vi "Wait till all GFG events stop_for fixed duration.vi"(8 "error in (no error)":errorcluster) -> (0 "error out":errorcluster)   [LabVIEW 2012]
doc: "SciScan 1.2 160622"
uses:
  <vilib>/Utility/VariantDataType/Type.ctl
  <vilib>/Utility/VariantDataType/VariantType.lvlib
panel:
  out "Array":T1(array[cluster])
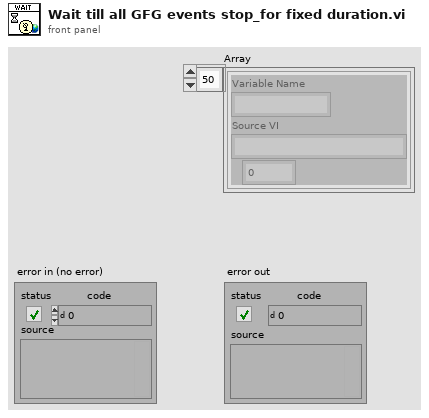
[diagram p1: front panel]
types:
  T1 = cluster{"Variable Name":string, "Source VI":string, u32}[]
  T2 = cluster{"Variable Name":string, "Source VI":string, u32}
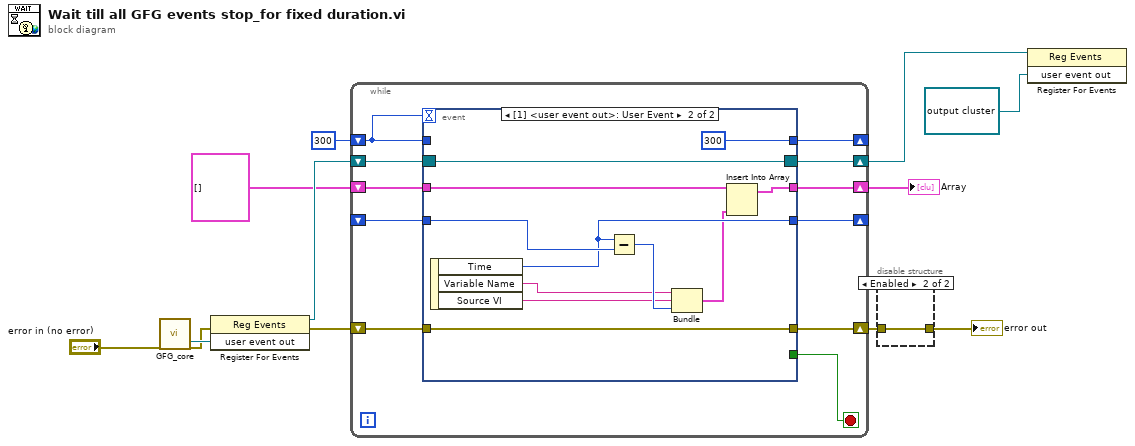
[diagram p0: block diagram]
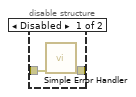
[diagram p2: hidden frame]
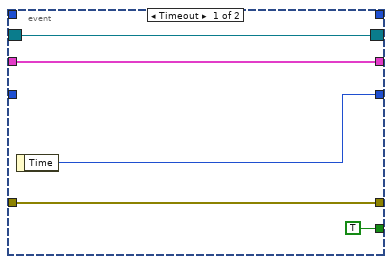
[diagram p3: hidden frame]
diagram:
  n1 = call "GFG_core.vi"("error in (no error)"="error in (no error)") -> ("user event out"=w2:refnum<user-event>, "error out"=w1:errorcluster)  [unwired: 12 in, 5 out]
  n2 = register-events(error in=w1, w2) -> (reference out=w12:refnum<event-registration>, error out=w9:errorcluster)  [unwired: 1 in]
  n3 = while {
    shift-right: [w22] -> _
    shift-left: 300 -> [w16]
    shift-right: [w20] -> _
    shift-left: _ -> [w19]
    shift-right: [w17] -> w6
    shift-left: w9 -> [w18]
    shift-right: [w15] -> w4
    shift-left: w12 -> [w23]
    shift-right: [w13] -> w7
    shift-left: T1 [] -> [w14]
    stop <- w21 stop-if-true
    n4 = event shown="[1] <user event out>: User Event" {
      selector: w23 -> [w26 w32]
      dyn-events: [w26 w32] -> w15
      timeout: w16 -> [_ _]
      tunnel: [_ 300] -> w22
      tunnel: [TRUE _] -> w21
      tunnel: [w25 w37] -> w20
      tunnel: w19 -> [_ w38]
      tunnel: w18 -> [w27 w35]
      tunnel: [w27 w35] -> w17
      tunnel: w16 -> [_ _]
      tunnel: w14 -> [w24 w31]
      tunnel: [w24 w29] -> w13
      event Timeout {
        n5 = event-data() -> ("Time"=w25:u32)  [unwired: 1 in]
      }
      event User Event {
        n6 = event-data() -> ("Time"=w37:u32, "Variable Name"=w33:string, "Source VI"=w34:string)  [unwired: 1 in]
        n7 = Subtract(x=w37, y=w38) -> (x-y=w36:u32)
        n8 = Bundle("Variable Name"=w33, "Source VI"=w34, w36) -> (w30:T2)  [unwired: 1 in]
        n9 = Insert Into Array(array=w31, new element=w30) -> (w29:T1)  [unwired: 1 in]
      }
    }
  }
  "Array" <- w7
  n10 = disable-structure shown="Enabled" {
    disable-tunnel: w6 -> [w41 w42]
    disable-tunnel: [w40 w42] -> w5
    frame Disabled {
      n11 = call <vilib>:"Simple Error Handler.vi"("error in (no error)"=w41) -> ("error out"=w40:errorcluster)  [unwired: 4 in, 4 out]
    }
    frame Enabled {
    }
  }
  "error out" <- w5
  n12 = register-events(reference=w4, refnum<user-event> refnum ("event source")) -> ()  [unwired: 1 in, 2 out]
